vi "GUI Timeout.vi"(7 "Timer States":T1, 8 "error in (no error)":errorcluster, 11 "Time to be inactive":i32) -> (0 "error out":errorcluster, 3 "Timeout":i32)   [LabVIEW 2017]
uses:
  Type Definitions/Timer States.ctl
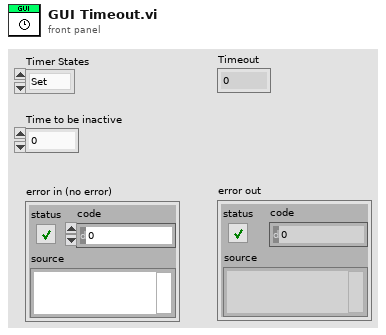
[diagram p1: front panel]
types:
  T1 = typedef "Timer States.ctl" = enum16{"Set", "Get"}
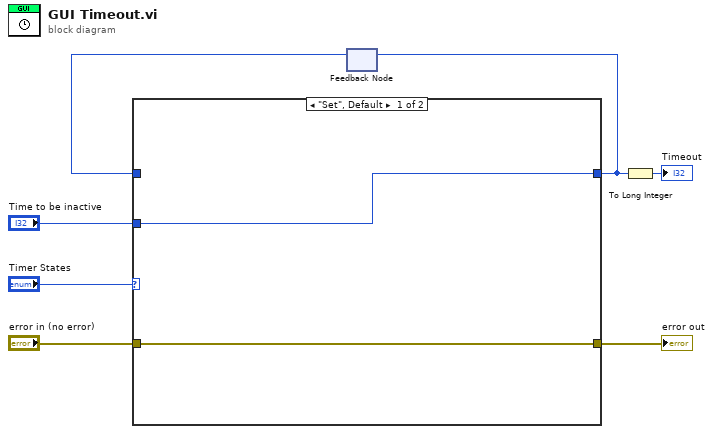
[diagram p0: block diagram]
diagram:
  n1 = feedback #1() -> (w5:i32)  [unwired: 1 in]
  n2 = case shown="\"Set\", Default" "Timer States" {
    tunnel: "error in (no error)" -> [w8 w10]
    tunnel: w5 -> [_ w11]
    tunnel: "Time to be inactive" -> [w9 _]
    tunnel: [w9 w11] -> w3
    tunnel: [w8 w10] -> w2
    frame "Set", Default {
    }
    frame "Get" {
    }
  }
  "error out" <- w2
  n3 = feedback-in #1(w3) -> ()
  n4 = To Long Integer(number=w3) -> (32bit integer=→"Timeout":i32)
